vi "teste centrage fonction.vi"() -> ()   [LabVIEW 2026]
uses:
  <vilib>/numeric/Random Number (Range) DBL.vi
  <vilib>/ptbypt/NI_PtbyPt.lvlib
panel:
  in  "x":dbl=100.0 format="%#_13g"
  in  "Model":T1(ring)=enum."sinus"
  in  "frequency sin X":dbl=2.0 caption="fréquence" format="%0.2f"
  in  "delta sin X":dbl=1000.0
  out "dt sin X":dbl=7.597
  in  "Enable":bool=TRUE caption="Activer"
  in  "Reset":bool caption="Réinitialisation"
  out "Histogram":dynamicdata(graph) caption="Histogramme"
  in  "stop":bool
  out "Graphe déroulant":cluster{dbl, i32}(graph)
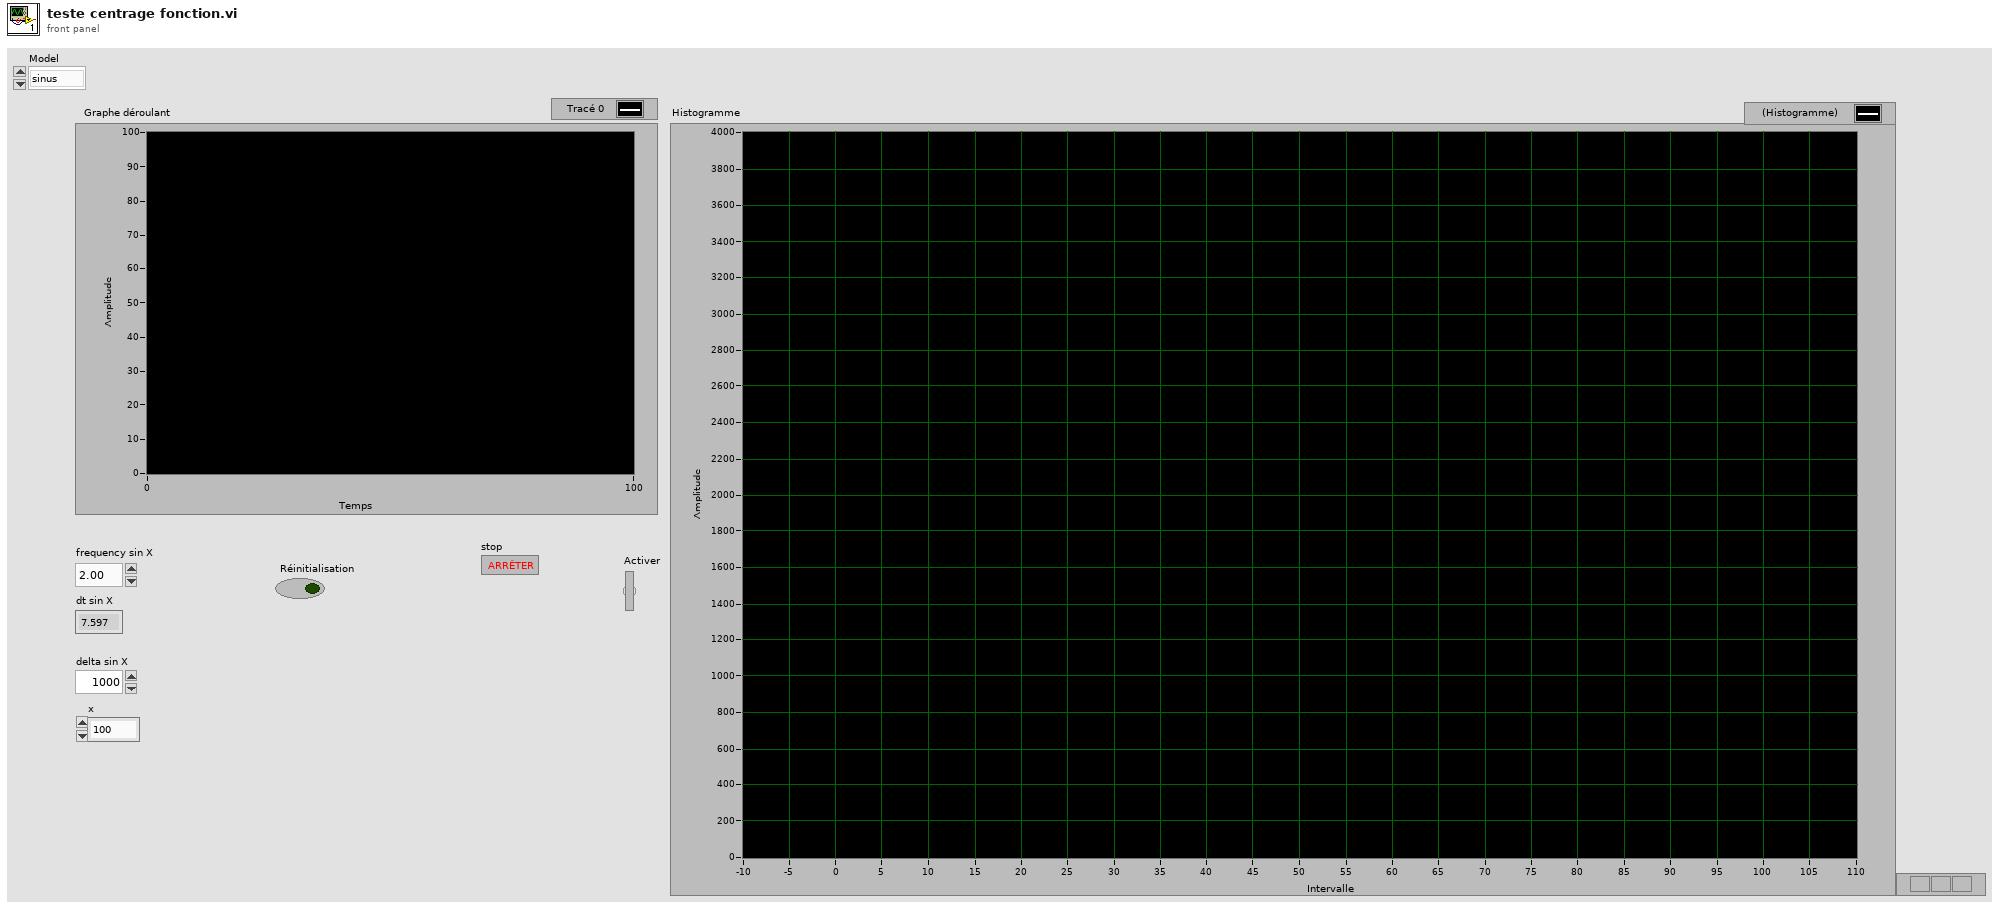
[diagram p1: front panel]
types:
  T1 = enum16{"initial", "aléatoire", "gaussien", "sinus"}
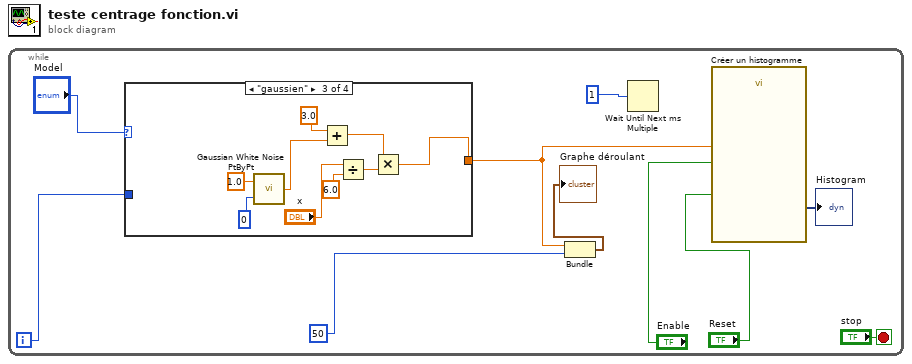
[diagram p0: block diagram]
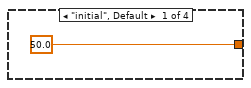
[diagram p2: hidden frame]
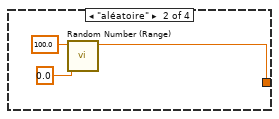
[diagram p3: hidden frame]
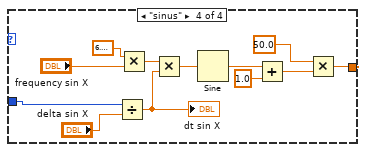
[diagram p4: hidden frame]
diagram:
  n1 = while {
    i -> [w1]
    stop <- "stop" stop-if-true
    n2 = case shown="\"gaussien\"" "Model" {
      tunnel: [50.0 ("number") w13 w15 w24] -> w2
      tunnel: w1 -> [_ _ _ w25]
      frame "initial", Default {
      }
      frame "aléatoire" {
        n3 = call-poly <vilib>:"Random Number (Range).vi"("lower bound (0)"=0.0, "upper bound (100)"=100.0) -> ("number"=w13:dbl)  [unwired: 9 in]
      }
      frame "gaussien" {
        n4 = call <vilib>:"Gaussian White Noise PtByPt.vi"("seed"=0, "standard deviation"=1.0) -> ("Gaussian white noise"=w21:dbl)  [unwired: 1 in]
        n5 = Add(x=3.0, y=w21) -> (x+y=w20:dbl)
        n6 = Divide(x="x", y=6.0) -> (x/y=w18:dbl)
        n7 = Multiply(x=w20, y=w18) -> (x*y=w15:dbl)
      }
      frame "sinus" {
        n8 = Divide(x=w25, y="delta sin X") -> (x/y=w32:dbl)
        "dt sin X" <- w32
        n9 = Multiply(x=6.283185307179586, y="frequency sin X") -> (x*y=w34:dbl)
        n10 = Multiply(x=w34, y=w32) -> (x*y=w31:dbl)
        n11 = Sine(x=w31) -> (sin(x)=w30:dbl)
        n12 = Add(x=w30, y=1.0) -> (x+y=w29:dbl)
        n13 = Multiply(x=50.0, y=w29) -> (x*y=w24:dbl)
      }
    }
    n14 = Bundle("number"=w2, 50) -> (→"Graphe déroulant":cluster{"number":dbl, i32})  [unwired: 1 in]
    n15 = Wait Until Next ms Multiple(millisecond multiple=u32 1 ("n millisecondes")) -> ()  [unwired: 1 out]
    n16 = call "Créer un histogramme"("Reset"="Reset", "Enable"="Enable", "Signal"=w2) -> ("Histogram"=→"Histogram":dynamicdata)  [unwired: 7 in, 1 out]
  }
